vi "Test Config Save.vi"() -> ()   [LabVIEW 2020, in "CDM-Config.lvlib"]
uses:
  CDM-Config.lvlib
  Config Manager/Config Manager.lvclass/Config Manager.ctl
  Config-JSON/Config-JSON.lvclass
  C:/dev/lv20CE/relink/lv-cdm/CDM-Config/Config Storage/Config Storage.lvclass
  Config Element/Set Owner.vi
  Config Element/Config Element.lvclass
  Config Storage/Config Storage.lvclass
  Config Manager/Config Manager.lvclass
panel:
  in  "Tree":string(tree)
  out "error out":errorcluster
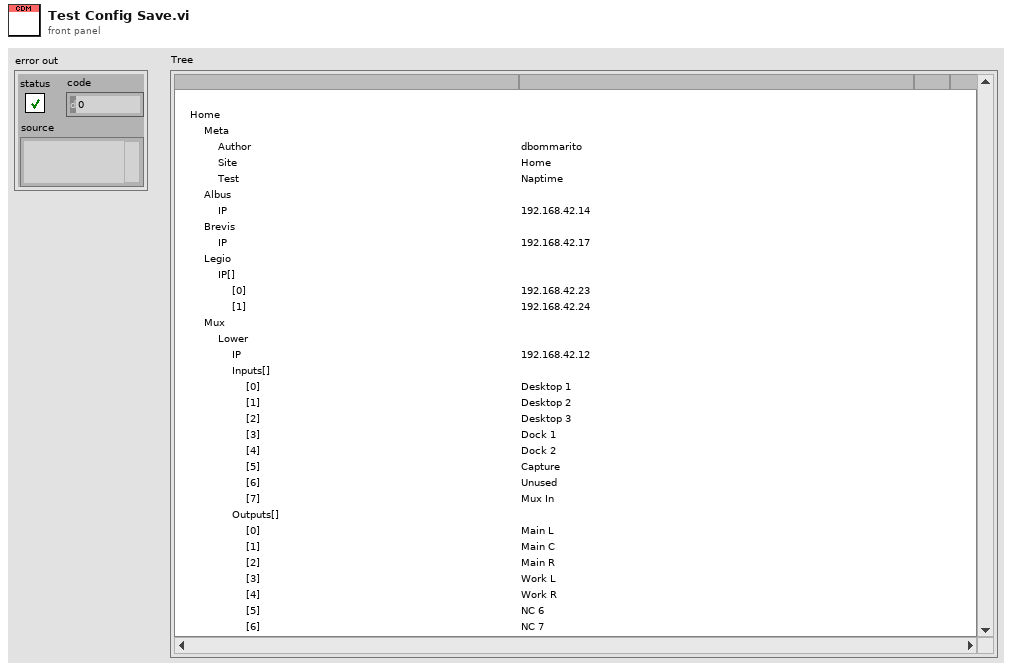
[diagram p1: front panel]
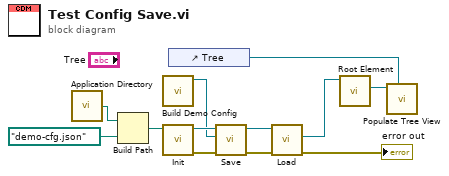
[diagram p0: block diagram]
diagram:
  n1 = call <vilib>:"Application Directory.vi"() -> ("Application Directory"=w9:path)
  n2 = Build Path(base path=w9, name or relative path=path "demo-cfg.json") -> (appended path=w11:path)
  n3 = call "Build Demo Config.vi"() -> ("Config Manager out"=w2:refnum<class "Config Manager.lvclass">)  [unwired: 11 in]
  n4 = call "Init.vi"("Path"=w11) -> ("error out"=w8:errorcluster, "Config-JSON out"=w10:refnum<class "Config-JSON.lvclass">)  [unwired: 9 in]
  n5 = control-ref of="Tree"() -> (w6:refnum<vi>)
  n6 = call "Save.vi"("error in (no error)"=w8, "Config"=w2, "Config Storage in"=w10) -> ("error out"=w5:errorcluster, "Config Storage out"=w4:refnum<class "Config-JSON.lvclass">)  [unwired: 7 in]
  n7 = call "Load.vi"("error in (no error)"=w5, "Config Storage in"=w4) -> ("error out"=→"error out":errorcluster, "Config"=w1:refnum<class "Config Manager.lvclass">)  [unwired: 7 in, 1 out]
  n8 = call "Root Element.vi"("Config Manager in"=w1) -> ("Root Element"=w7:refnum<class "Config Element.lvclass">)  [unwired: 8 in, 2 out]
  n9 = call "Populate Tree View.vi"("Tree"=w6, "Element"=w7) -> ()  [unwired: 9 in, 1 out]
